vi "Bunde ROI info.vi"(0 "ROI Coordinates":i32[](array[numeric]), 1 "ROI Enum":T2, 2 "Zoom":dbl, 3 "ZplaneIndex":i32, 7 "Zplanecode":u8) -> (14 "ROI Info":T1={"Coordinates"=[], "Zoom"=1.0, "ROI Enum"=enum."Point", "Z planeIdx(s)"=[], "Z planecodes(s)"=[], "Z start"=0.0, "Z stop"=0.0} {"Zoom" min=1.0 max=10.0 step=0.10000000149011612})   [LabVIEW 2017]
uses:
  Typedefs/ROI ID Enum.ctl
  Typedefs/ROI spec.ctl
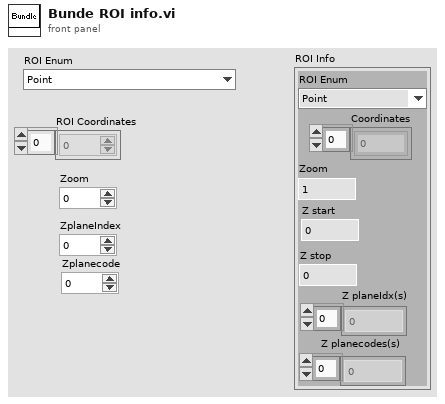
[diagram p1: front panel]
types:
  T1 = typedef "ROI spec.ctl" = cluster{"Coordinates":i32[], "Zoom":dbl, "ROI Enum":T2, "Z planeIdx(s)":i32[], "Z planecodes(s)":u8[], "Z start":dbl, "Z stop":dbl}
  T2 = typedef "ROI ID Enum.ctl" = enum16{"Point", "MiniScan", "Comp. MiniScan", "Rectangle", "Comp. volume", "Arb. plane point"}
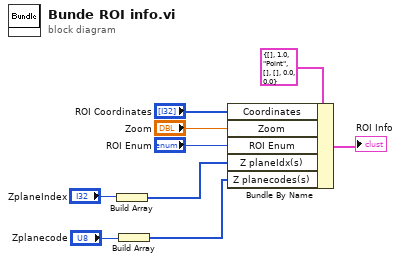
[diagram p0: block diagram]
diagram:
  n1 = Build Array("ZplaneIndex") -> (w4:i32[])
  n2 = Build Array("Zplanecode") -> (w1:u8[])
  n3 = Bundle By Name(cluster=T1 {"Coordinates"=[], "Zoom"=1.0, "ROI Enum"=enum."Point", "Z planeIdx(s)"=[], "Z planecodes(s)"=[], "Z start"=0.0, "Z stop"=0.0} ("input cluster"), "Coordinates"="ROI Coordinates", "Zoom"="Zoom", "ROI Enum"="ROI Enum", "Z planeIdx(s)"=w4, "Z planecodes(s)"=w1) -> (→"ROI Info":T1)
